vi "PicoScope2000aExampleStreamingMSO.vi"() -> ()   [LabVIEW 2010]
doc: "This example demonstrates how to use the PicoScope Labview library to stream data from a PicoScope 2000 Series Device"
uses:
  <vilib>/Waveform/DWDTOps.llb/DWDT Analog to Digital.vi
  PicoScope2000aLib/PicoScope2000aAnalogChannelSettings.ctl
  PicoScope2000aLib/PicoScope2000aDigitalChannelSettings.ctl
panel:
  in  "Write to TDMS":bool
  in  "Port 0 Settings":T1={"Enabled"=FALSE, "Logic Level"=9830} {"Logic Level" items=["1.5V TTL"=9830, "2.5V CMOS"=16383]}
  in  "Channel A Settings":T2={"Enabled"=TRUE, "Coupling"=1, "Range"=6, "Analogue Offset"=0.0} {"Analogue Offset" format="%#_6p"; "Range" items=["20 mV"=1, "50 mV"=2, "100 mV"=3, "200 mV"=4, "500 mV"=5, "1 V"=6, "2 V"=7, "5 V"=8, "10 V"=9, "20 V"=10]; "Coupling" items=["AC", "DC"]}
  out "Analog Channels":T3(graph)
  out "Raw Sample Interval (sec)":dbl=1.0000000130088963e-06 format="%#.5p"
  out "Max ADC value":i16
  out "Chunk time (ms)":u32
  out "Elapsed time":dbl
  in  "Data file":path=path "PicoScope2000aExampleStreaming ChA Data"
  out "size(s)":i32
  out "Queue depth":i32(graph)
  out "queue depth":i32
  in  "Buffer and Transfer Settings":T4={"startIndex"=0, "Samples"=1000000, "Down Sample Ratio"=1, "Down-Sample Mode"=0} {"Down-Sample Mode" items=["None"=0, "Aggregate"=1, "Decimate"=2, "Average"=4]; "Down Sample Ratio" step=1; "Samples" format="%_6p"}
  out "TriggeredAt (In Buffer)":u32 format="%#.6p"
  out "TriggeredAt (Total samples)":u32 format="%#.6p"
  in  "Acquisition Settings":T5={"Auto Stop"=TRUE, "Desired Sample Interval"=1, "Pre-trigger Samples"=0, "Post-trigger Samples"=1000000, "Down-Sample Ratio"=1, "Down-Sample Mode"=0, "Time Units"=3} {"Time Units" items=["Nanoseconds (ns)"=2, "Microseconds (us)"=3, "Milliseconds (ms)"=4, "Seconds (s)"=5]; "Down-Sample Mode" items=["None"=0, "Aggregate"=1, "Decimate"=2, "Average"=4]; "Post-trigger Samples" format="%#.6p"; "Pre-trigger Samples" format="%#_6p"}
  out "Port 0":digitalwaveform(graph)={"t0"=timestamp(0 s since 1904-01-01), "dt"=1.0000000130088963e-06, "Y"={"transitions"=[], "data"=[]}}
  in  "Trigger Settings":T6={"Trigger Enabled"=FALSE, "Trigger Source"=enum."Channel A", "Trigger Threshold (volts)"=0.0, "Trigger Direction"=2, "Trigger Delay (samples)"=0, "Auto Trigger Time (ms)"=1000} {"Trigger Direction" items=["Rising"=2, "Falling"=3]}
  out "Triggered":bool
  out "DownSample Interval (sec)":dbl=1.0000000130088963e-06 format="%#.5p"
  out "Total Samples":u32 format="%#.6p"
  out "Auto Stopped":bool
  in  "Serial Number":string
  in  "Open Using Serial Number":bool
  out "Number of Samples per Capture":u32 format="%#.6p"
  in  "Apply  Settings":bool
  in  "stop":bool
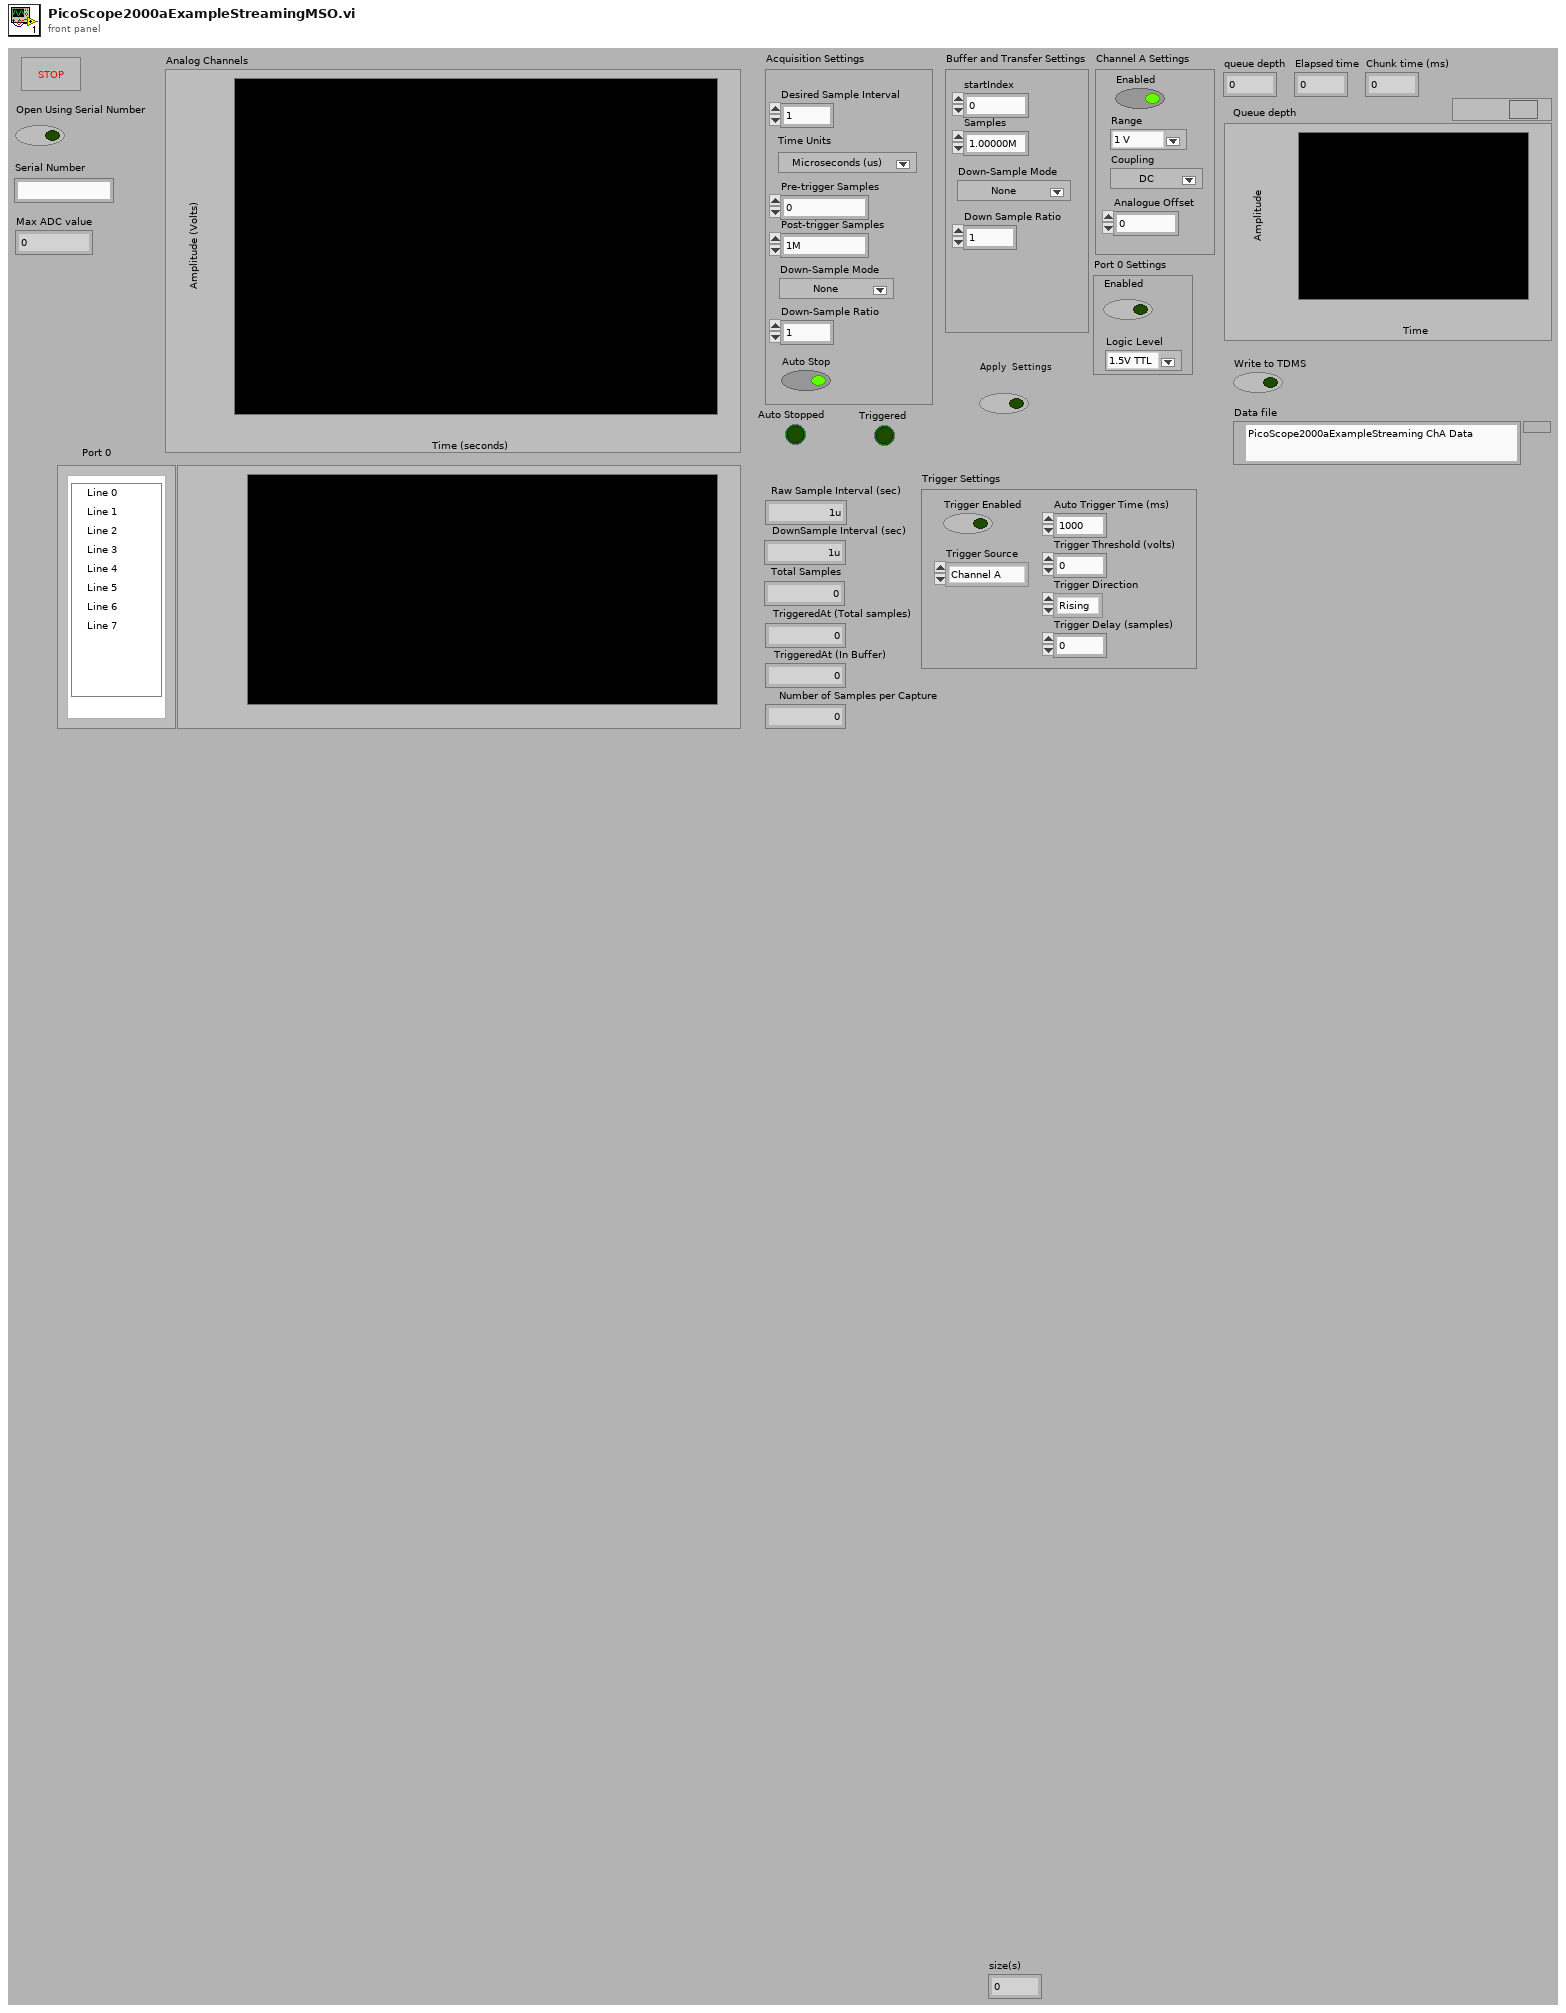
[diagram p1: front panel]
types:
  T1 = typedef "PicoScope2000aDigitalChannelSettings.ctl" = cluster{"Enabled":bool, "Logic Level":i16}
  T2 = typedef "PicoScope2000aAnalogChannelSettings.ctl" = cluster{"Enabled":bool, "Coupling":i16, "Range":u32, "Analogue Offset":sgl}
  T3 = cluster{i32, "DownSample Interval (sec)":dbl, "Data":dbl[]}
  T4 = cluster{"startIndex":u64, "Samples":u64, "Down Sample Ratio":u64, "Down-Sample Mode":u32}
  T5 = cluster{"Auto Stop":bool, "Desired Sample Interval":u32, "Pre-trigger Samples":u32, "Post-trigger Samples":u32, "Down-Sample Ratio":u32, "Down-Sample Mode":i32, "Time Units":u32}
  T6 = cluster{"Trigger Enabled":bool, "Trigger Source":enum16{"Channel A", "Channel B", "Channel C", "Channel D", "Ext."}, "Trigger Threshold (volts)":dbl, "Trigger Direction":u16, "Trigger Delay (samples)":u32, "Auto Trigger Time (ms)":i16}
  T7 = enum16{"open", "open or create", "create or replace", "create", "open (read-only)"}
  T8 = cluster{"Driver Version":string, "USB Version":string, "Hardware":string, "Variant":string, "Batch and Serial":string, "Cal Date":string, "Kernel Version":string, "Digital HW Version":string, "Analogue HW Version":string, "Firmware 1":string, "Firmware 2":string, "MSO":bool, "Number of Channels":i16}
  T9 = cluster{"Channel A Buffer":i16[], "Channel B Buffer":i16[], "Channel C Buffer":i16[], "Channel D Buffer":i16[], "Channel E Buffer":i16[], "Channel F Buffer":i16[], "Channel G Buffer":i16[], "Channel H Buffer":i16[], "Port 0":i16[], "Port 1":i16[]}
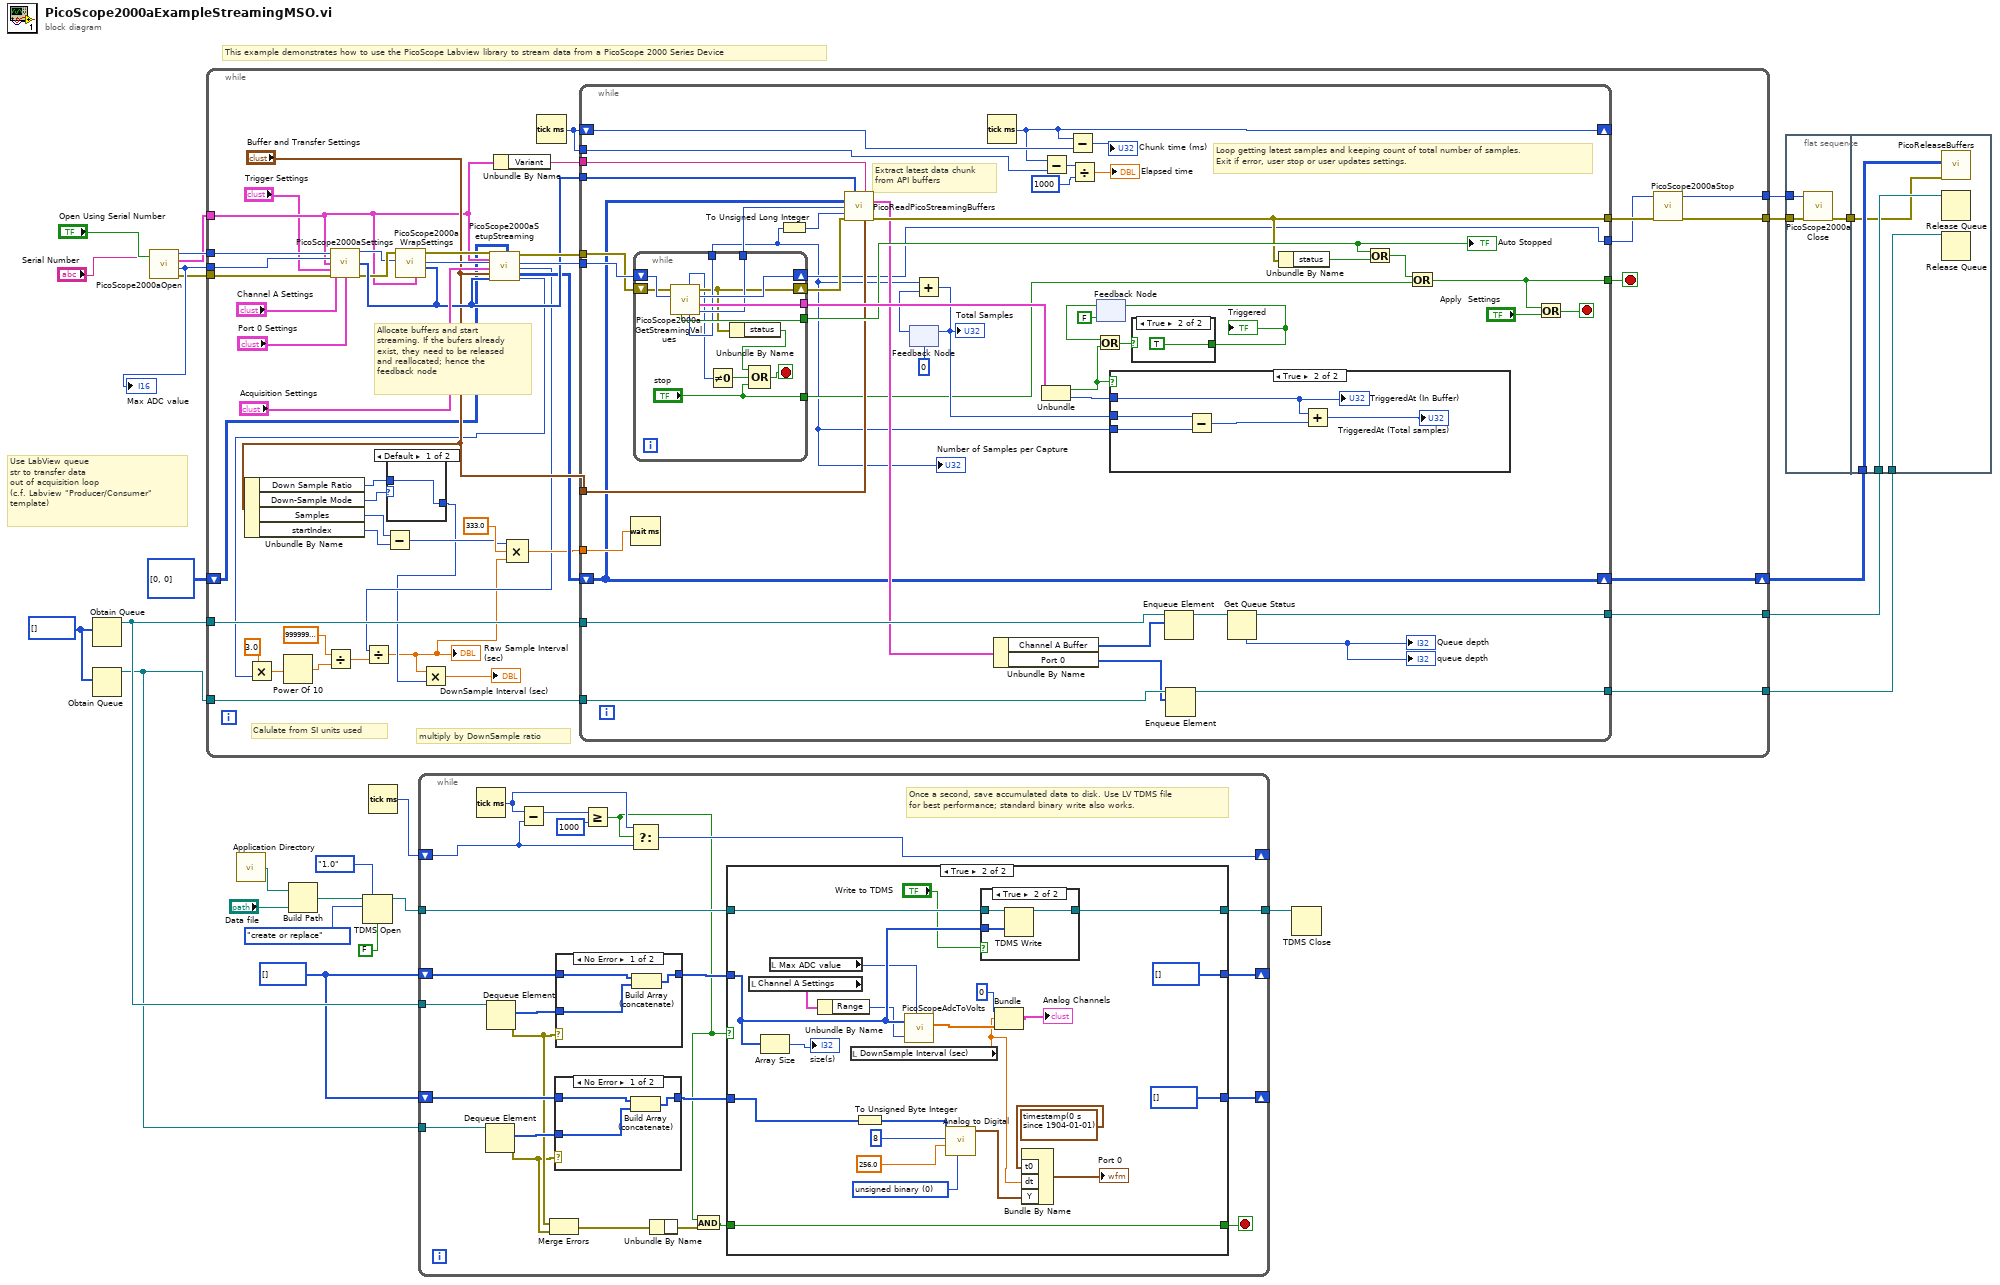
[diagram p0: block diagram]
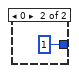
[diagram p6: hidden frame]
diagram:
  w14 = i16[] [] ("History Data")
  w17 = i16[] [] ("History Data")
  # "Use LabView queue\nstr to transfer data\nout of acquisition loop\n(c.f. Labview \"Producer/Consumer\"\ntemplate)"
  # "This example demonstrates how to use the PicoScope Labview library to stream data from a PicoScope 2000 Series Device"
  n1 = Obtain Queue(element data type=w17) -> (queue out=w26:refnum<queue>)  [unwired: 4 in, 2 out]
  n2 = Obtain Queue(element data type=w17) -> (queue out=w15:refnum<queue>)  [unwired: 4 in, 2 out]
  n3 = call "PicoScope2000aOpen.vi"("Serial Number"="Serial Number", "Use Serial Number"="Open Using Serial Number") -> ("error out"=w5:errorcluster, "Max Adc value"=w6:i16, "Device Info"=w3:T8, "handle"=w4:i16)  [unwired: 4 in, 2 out]
  "Max ADC value" <- w6
  n4 = while {
    tunnel: [w56] -> w25
    tunnel: w6 -> [w31]
    tunnel: [w63] -> w24
    tunnel: w26 -> [w62]
    tunnel: [w60] -> w16
    tunnel: w15 -> [w59]
    tunnel: [w37] -> w8
    tunnel: w5 -> [w35]
    tunnel: w4 -> [w34]
    tunnel: w3 -> [w30]
    shift-right: [w28] -> w2
    shift-left: u64[][] [[0], [0]] ("Pointer array") -> [w27]
    stop <- w73 stop-if-true
    # "Allocate buffers and start\nstreaming. If the bufers already\nexist, they need to be released\nand reallocated; hence the\nfeedback node"
    # "Calulate from SI units used"
    # "multiply by DownSample ratio"
    n5 = Unbundle By Name("Buffer and Transfer Settings") -> ("Down Sample Ratio"=w67:u64, "Down-Sample Mode"=w68:u32, "Samples"=w53:u64, "startIndex"=w52:u64)
    n6 = call "PicoScope2000aSettings.vi"("handle in"=w34, "Channel A Settings"="Channel A Settings", "Max_adc"=w31, "Device Info"=w30, "Trigger Settings"="Trigger Settings", "error in"=w35, "Port 0 Settings"="Port 0 Settings") -> ("handle out"=w32:i16, "Enabled Array"=w65:i16[], "error out"=w36:errorcluster)  [unwired: 6 in]
    n7 = Subtract(x=w53, y=w52) -> (x-y=w42:u64)
    n8 = case shown="Default" w68 {
      tunnel: [w74 u32 1 ("Down-Sample Ratio")] -> w40
      tunnel: w67 -> [w74 _]
      frame Default {
      }
      frame 0 {
      }
    }
    n9 = call "PicoScope2000aWrapSettings.vi"("Device Info"=w30, "Enabled array"=w65, "Handle In"=w32, "error in (no error)"=w36) -> ("Handle Out"=w70:i16, "error out"=w69:errorcluster)  [unwired: 6 in]
    n10 = call "PicoScope2000aSetupStreaming.vi"("error in"=w69, "Device Info"=w30, "handle in"=w70, "Acquisition Settings"="Acquisition Settings", "Buffer and Transfer Settings"="Buffer and Transfer Settings", "enabled array"=w65, "Pointers In"=w27) -> ("Pointer array"=w61:u64[][], "error out"=w71:errorcluster, "handle out"=w72:i16, "Sample Interval"=w41:u32, "sampleIntervalTimeUnits"=w44:u32)  [unwired: 8 in]
    n11 = Multiply(x=3.0, y=w44) -> (x*y=w51:dbl)
    n12 = Power Of 10(x=w51) -> (10^x=w50:dbl)
    n13 = Divide(x=sgl 1000000000000000.0 ("y"), y=w50) -> (x/y=w49:dbl)
    n14 = Divide(x=w41, y=w49) -> (x/y=w39:dbl)
    "Raw Sample Interval (sec)" <- w39
    n15 = Multiply(x=w39, y=w40) -> (x*y=→"DownSample Interval (sec)":dbl)
    n16 = Unbundle By Name(w30) -> ("Variant"=w38:string)
    n17 = Compound Arithmetic op=MULTIPLY(w42, 333.0 ("value"), w39) -> (w45:dbl)
    n18 = Tick Count (ms)() -> (millisecond timer value=w54:u32)
    n19 = while {
      tunnel: [w88] -> w55
      tunnel: [w120] -> w73
      tunnel: w72 -> [w105]
      tunnel: w71 -> [w104]
      tunnel: [w101] -> w57
      tunnel: "Buffer and Transfer Settings" -> [w103]
      tunnel: w65 -> [w100]
      tunnel: [w98] -> w63
      tunnel: w62 -> [w96]
      shift-right: [w90] -> _
      shift-left: w54 -> [w91]
      tunnel: w38 -> [w85]
      tunnel: [w76] -> w60
      tunnel: w59 -> [w84]
      tunnel: w54 -> [w79]
      tunnel: w45 -> [w78]
      shift-right: [w77] -> w28
      shift-left: w61 -> [w77]
      stop <- w119 stop-if-true
      # "Loop getting latest samples and keeping count of total number of samples. \nExit if error, user stop or user updates settings."
      # "Extract latest data chunk\nfrom API buffers"
      n20 = Wait (ms)(milliseconds to wait=w78) -> ()  [unwired: 1 out]
      n21 = while {
        tunnel: [w134] -> w118
        tunnel: [w133] -> w115
        tunnel: [w129] -> w86
        tunnel: [w128] -> w80
        shift-right: [w130] -> w88
        shift-left: w105 -> [w132]
        shift-right: [w127] -> w102
        shift-left: w104 -> [w131]
        tunnel: ["stop"] -> w82
        stop <- w123 stop-if-true
        n22 = call "PicoScope2000aGetStreamingValues.vi"("handle in"=w132, "error in"=w131) -> ("Start Index"=w129:u32, "Trigger"=w134:cluster{bool, "triggeredAt":u32}, "handle out"=w130:i16, "error out"=w127:errorcluster, "Number of Samples"=w128:i32, "ready"=w126:i16, "Auto Stopped"=w133:bool)  [unwired: 3 in]
        n23 = Not Equal To 0?(x=w126) -> (x != 0?=w124:bool)
        n24 = Unbundle By Name(w127) -> ("status"=w125:bool)
        n25 = Compound Arithmetic op=OR(w125, w124, "stop") -> (w123:bool)
      }
      "Number of Samples per Capture" <- w80
      "Auto Stopped" <- w115
      n26 = To Unsigned Long Integer(number=w80) -> (unsigned 32bit integer=w81:u32)
      n27 = call "PicoReadPicoStreamingBuffers.vi"("enabled array"=w100, "Buffer and Transfer Settings"=w103, "Variant"=w85, "Pointer array"=w77, "Offset Index"=w86, "Number of Samples"=w81, "error in (no error)"=w102) -> ("Buffers (Max or non-aggregated)"=w95:T9, "error out"=w101:errorcluster)  [unwired: 6 in, 1 out]
      n28 = feedback #1(u32 0) -> (w111:u32)
      n29 = Add(x=w80, y=w111) -> (x+y=w109:u32)
      "Total Samples" <- w109
      n30 = feedback-in #1(w109) -> ()
      n31 = Tick Count (ms)() -> (millisecond timer value=w90:u32)
      n32 = Unbundle By Name(w95) -> ("Channel A Buffer"=w87:i16[], "Port 0"=w83:i16[])
      n33 = Subtract(x=w90, y=w79) -> (x-y=w94:u32)
      n34 = Unbundle(w118) -> (w107:bool, "triggeredAt"=w106:u32)
      n35 = Subtract(x=w90, y=w91) -> (x-y=→"Chunk time (ms)":u32)
      n36 = Divide(x=w94, y=u32 1000) -> (x/y=→"Elapsed time":dbl)
      n37 = feedback #2(FALSE) -> (w113:bool)
      n38 = Or(x=w113, y=w107) -> (x .or. y?=w110:bool)
      n39 = case shown="True" w107 {
        tunnel: w80 -> [_ w135]
        tunnel: w109 -> [_ w139]
        tunnel: w106 -> [_ w137]
        frame False {
        }
        frame True {
          n40 = Subtract(x=w139, y=w135) -> (x-y=w138:u32)
          n41 = Add(x=w137, y=w138) -> (x+y=→"TriggeredAt (Total samples)":u32)
          "TriggeredAt (In Buffer)" <- w137
        }
      }
      n42 = case shown="True" w110 {
        selector: w110 -> [w140 _]
        tunnel: [w140 TRUE] -> w108
        frame False {
        }
        frame True {
        }
      }
      "Triggered" <- w108
      n43 = feedback-in #2(w108) -> ()
      n44 = Enqueue Element(queue=w96, element=w87) -> (queue out=w97:refnum<queue>)  [unwired: 2 in, 2 out]
      n45 = Enqueue Element(queue=w84, element=w83) -> (queue out=w76:refnum<queue>)  [unwired: 2 in, 2 out]
      n46 = Get Queue Status(queue=w97) -> (queue out=w98:refnum<queue>, # elements in queue=→"queue depth" →"Queue depth":i32)  [unwired: 2 in, 6 out]
      n47 = Unbundle By Name(w101) -> ("status"=w117:bool)
      n48 = Or(x=w115, y=w117) -> (x .or. y?=w116:bool)
      n49 = Or(x=w116, y=w82) -> (x .or. y?=w120:bool)
      n50 = Or(x=w120, y="Apply  Settings") -> (x .or. y?=w119:bool)
    }
    n51 = call "PicoScope2000aStop.vi"("error in (no error)"=w57, "handle in"=w55) -> ("error out"=w37:errorcluster, "handle out"=w56:i16)  [unwired: 8 in]
  }
  n52 = call <vilib>:"Application Directory.vi"() -> ("Application Directory"=w11:path)
  n53 = Build Path(base path=w11, name or relative path="Data file") -> (appended path=w12:path)
  n54 = TDMS Open(6:FALSE ("disable buffering? (T)"), 7:enum16{"1.0", "2.0"}."1.0" ("file format version (2.0)"), 10:T7."create or replace" ("operation (0:open)"), 11:w12) -> (3:w21:refnum<k34>)  [unwired: 2 in, 1 out]
  n55 = Tick Count (ms)() -> (millisecond timer value=w23:u32)
  n56 = while {
    tunnel: w26 -> [w164]
    shift-right: [w156] -> _
    shift-left: w14 -> [w163]
    shift-right: [w158] -> _
    shift-left: w23 -> [w159]
    tunnel: w21 -> [w155]
    tunnel: [w154] -> w20
    tunnel: w15 -> [w152]
    shift-right: [w149] -> _
    shift-left: w14 -> [w151]
    stop <- w144 stop-if-true
    # "Once a second, save accumulated data to disk. Use LV TDMS file\nfor best performance; standard binary write also works."
    n57 = Tick Count (ms)() -> (millisecond timer value=w160:u32)
    n58 = Dequeue Element(queue=w152) -> (element=w153:i16[], error out=w147:errorcluster)  [unwired: 2 in, 2 out]
    n59 = Dequeue Element(queue=w164) -> (element=w165:i16[], error out=w148:errorcluster)  [unwired: 2 in, 2 out]
    n60 = Subtract(x=w160, y=w159) -> (x-y=w162:u32)
    n61 = Merge Errors(w148, w147) -> (w146:errorcluster)
    n62 = case shown="No Error" w147 {
      tunnel: w151 -> [w168 w169]
      tunnel: [w167 w169] -> w150
      tunnel: w153 -> [w166 _]
      frame No Error {
        n63 = Build Array (concatenate)(w168, w166) -> (w167:i16[])
      }
      frame Error {
      }
    }
    n64 = case shown="No Error" w148 {
      tunnel: w163 -> [w203 w204]
      tunnel: [w202 w204] -> w157
      tunnel: w165 -> [w201 _]
      frame No Error {
        n65 = Build Array (concatenate)(w203, w201) -> (w202:i16[])
      }
      frame Error {
      }
    }
    n66 = Greater Or Equal?(x=w162, y=u32 1000) -> (x >= y?=w145:bool)
    n67 = Select(t=w160, s=w145, f=w159) -> (s? t:f=w158:u32)
    n68 = And(x=w145) -> (y=w142:errorcluster, x .and. y?=w143:bool)
    n69 = Unbundle By Name(w146, w142) -> ()
    n70 = case shown="True" w145 {
      tunnel: w157 -> [w173 w192]
      tunnel: [w173 i16[] [] ("History Data")] -> w156
      tunnel: w155 -> [w172 w194]
      tunnel: [w172 w193] -> w154
      tunnel: w150 -> [w171 w179]
      tunnel: [w171 i16[] [] ("History Data")] -> w149
      tunnel: [w170 w175] -> w144
      tunnel: w143 -> [w170 w175]
      frame False {
      }
      frame True {
        w185 = u16 0 items=["unsigned binary", "offset binary", "2's complement"] ("data format (offset binary)")
        n71 = local read "Channel A Settings"() -> (w176:T2)
        n72 = Array Size(array=w192) -> (size(s)=→"size(s)":i32)
        n73 = local read "Max ADC value"() -> (w188:i16)
        n74 = Unbundle By Name(w176) -> ("Range"=w191:u32)
        n75 = local read "DownSample Interval (sec)"() -> (w180:dbl)
        n76 = To Unsigned Byte Integer(number=w179) -> (unsigned 8bit integer=w184:u8[])
        n77 = call "PicoScopeAdcToVolts.vi"("Max_adc"=w188, "Range Index"=w191, "Data"=w192) -> ("Data"=w189:dbl[])
        n78 = call-poly <vilib>:"Analog to Digital.vi"("data format (offset binary)"=w185, "full-scale range (pk-pk)"=256.0, "resolution (16 bit)"=8, "analog waveform"=w184) -> ("digital waveform"=w181:digitalwaveform)  [unwired: 4 in, 3 out]
        n79 = case shown="True" "Write to TDMS" {
          tunnel: w194 -> [w197 w200]
          tunnel: [w197 w199] -> w193
          tunnel: w192 -> [_ w198]
          frame False {
          }
          frame True {
            n80 = TDMS Write(0:w200, 9:w198) -> (4:w199:refnum<k34>)  [unwired: 4 in, 3 out]
          }
        }
        n81 = Bundle(0, "DownSample Interval (sec)"=w180, "Data"=w189) -> (→"Analog Channels":T3)  [unwired: 1 in]
        n82 = Bundle By Name("t0"=timestamp(0 s since 1904-01-01), "dt"=w180, "Y"=w181) -> (→"Port 0":digitalwaveform)  [unwired: 1 in]
      }
    }
  }
  n83 = TDMS Close(11:w20) -> ()  [unwired: 1 in, 2 out]
  n84 = flat-sequence {
    tunnel: w25 -> [w207]
    tunnel: w8 -> [w206]
    tunnel: [w205] -> w7
    tunnel: w2 -> [w211]
    tunnel: w24 -> [w210]
    tunnel: w16 -> [w209]
    tunnel: w7 -> [w208]
    frame #0 {
      n85 = call "PicoScope2000aClose.vi"("error in (no error)"=w206, "handle in"=w207) -> ("error out"=w205:errorcluster)  [unwired: 8 in, 1 out]
    }
    frame #1 {
      n86 = call "PicoReleaseBuffers.vi"("error in (no error)"=w208, "Pointer array"=w211) -> ()  [unwired: 8 in, 2 out]
      n87 = Release Queue(queue=w210) -> ()  [unwired: 2 in, 3 out]
      n88 = Release Queue(queue=w209) -> ()  [unwired: 2 in, 3 out]
    }
  }
